vi "Close Instrument.vi"(8 "error in (no error)":errorcluster, 11 "VoltageUpdate":refnum<class "VoltageUpdate.lvclass">) -> (0 "error out":errorcluster, 3 "VoltageUpdate out":refnum<class "VoltageUpdate.lvclass">)   [LabVIEW 2016, in "VoltageUpdate.lvclass"]
uses:
  VoltageUpdate.lvclass
  VoltageUpdate.lvclass/VoltageUpdate.ctl
  <userlib>/LevyLab/Levylab Instruments/Instrument Types/VSource/Instrument.VSource.lvclass
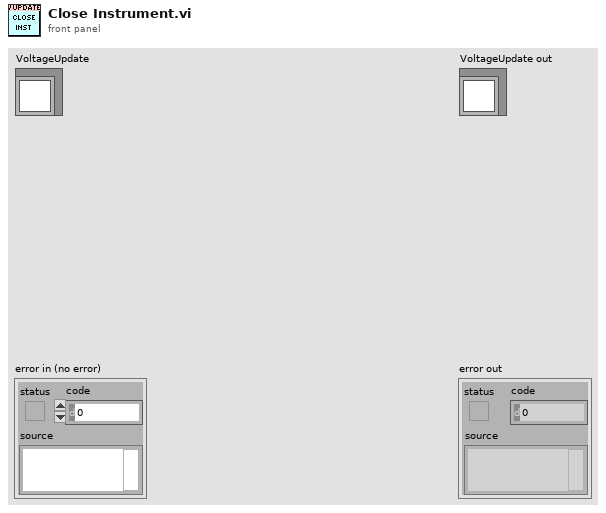
[diagram p1: front panel]
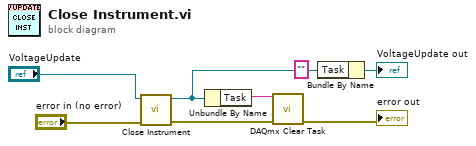
[diagram p0: block diagram]
diagram:
  n1 = call-parent "Close Instrument.vi"("error in (no error)"="error in (no error)", "Instrument in"="VoltageUpdate") -> ("error out"=w1:errorcluster, "Instrument out"=w5:refnum<class "VoltageUpdate.lvclass">)  [unwired: 8 in]
  n2 = Unbundle By Name(w5) -> ("Task"=w6:string)
  n3 = call <vilib>:"DAQmx Clear Task.vi"("task in"=w6, "error in"=w1) -> ("error out"=→"error out":errorcluster)  [unwired: 13 in]
  n4 = Bundle By Name(cluster=w5, "Task"="") -> (→"VoltageUpdate out":refnum<class "VoltageUpdate.lvclass">)
